vi "Actor Core.vi"(8 "error in":errorcluster, 11 "Example Sink in":refnum<class "Example Sink.lvclass">) -> (0 "error out":errorcluster, 3 "Actor out":refnum<class "Actor.lvclass">)   [LabVIEW 2020, in "Example Sink.lvlib" / "Example Sink.lvclass"]
doc: "(<B>Filename</B>: Actor Framework.lvlib:Actor.lvclass:Actor Core.vi)\n\nReceives messages to the actor, reacts to them, and initiates any error handling that may shut the actor down.\n\nDescendant classes may override this VI to append parallel tasks for the actor to complete while it handles messages. Overrides use the Call Parent Class Method node."
uses:
  Example Sink.lvclass
  <vilib>/ActorFramework/Actor/Actor.lvclass
  Example Sink.lvclass/Example Sink.ctl
panel:
  out "String":string
  out "Waveform Graph":dbl[](graph)
  out "Gauge":T1(knob)={"Numeric"=0.0, "Numeric"=10.76717224956633, "Numeric"=10.76717224956633} scale=0.0..12.0
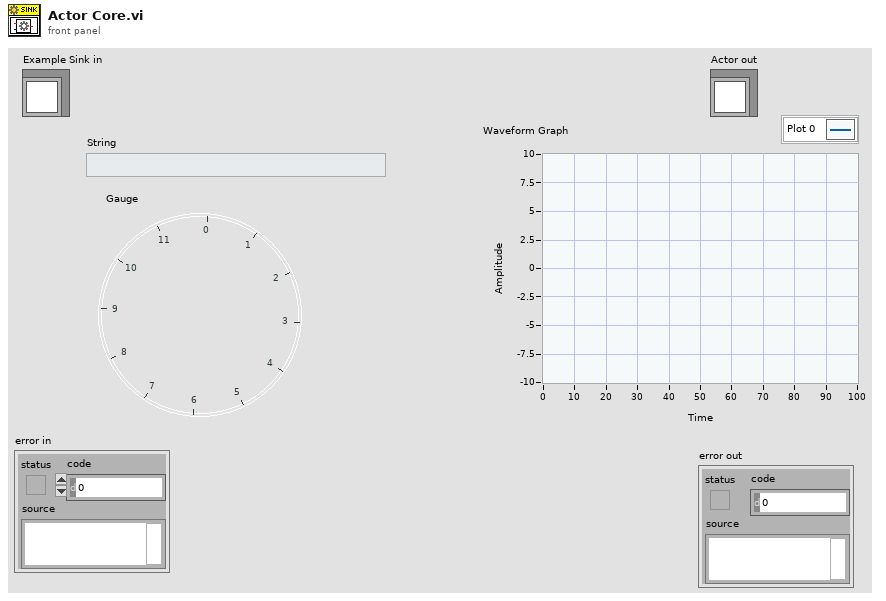
[diagram p1: front panel]
types:
  T1 = cluster{"Numeric":dbl, "Numeric":dbl, "Numeric":dbl}
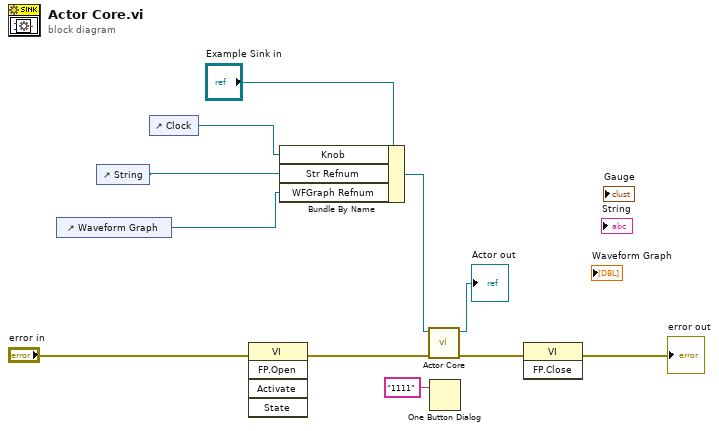
[diagram p0: block diagram]
diagram:
  n1 = control-ref of="Waveform Graph"() -> (w7:refnum<vi>)
  n2 = control-ref of="String"() -> (w6:refnum<vi>)
  n3 = control-ref of="Clock"() -> (w8:refnum<vi>)
  n4 = invoke class="VI" method="FP.Open"(error in="error in") -> (error out=w4:errorcluster)  [unwired: 4 in, 4 out]
  n5 = Bundle By Name(cluster="Example Sink in", "Knob"=w8, "Str Refnum"=w6, "WFGraph Refnum"=w7) -> (w9:refnum<class "Example Sink.lvclass">)
  n6 = call-parent "Actor Core.vi"("error in"=w4, "Actor in"=w9) -> ("error out"=w3:errorcluster, "Actor out"=→"Actor out":refnum<class "Actor.lvclass">)  [unwired: 8 in]
  n7 = One Button Dialog(message="1111") -> ()  [unwired: 1 in, 1 out]
  n8 = invoke class="VI" method="FP.Close"(error in=w3) -> (error out=→"error out":errorcluster)  [unwired: 2 in, 2 out]
